vi "Get Result.vi"(8 "error in (no error)":errorcluster, 11 "LR-700 in":refnum<class "Linear Research.lvclass">) -> (0 "error out":errorcluster, 2 "Mag Lab Result.lvclass":refnum<class "Mag Lab Result.lvclass">, 3 "LR-700 out":refnum<class "Linear Research.lvclass">)   [LabVIEW 2015, in "Linear Research.lvclass"]
uses:
  Linear Research.lvclass
  Mag Lab Result/Mag Lab Result.lvclass
  Linear Research Parameters.ctl
  Mag Lab Hardware.lvclass/Mag Lab Hardware.ctl
  Mag Lab Root/Mag Lab Root.lvclass/Mag Lab Root.ctl
  Linear Research.lvclass/Linear Research.ctl
  Mag Lab Result/Mag Lab Result.lvclass/Mag Lab Result.ctl
  Mag Lab Properties/Mag Lab Parameters.lvclass
  Mag Lab Hardware.lvclass
  Mag Lab Error Handler/Mag Lab Error Handler.lvclass
  Mag Lab Root/Mag Lab Root.lvclass
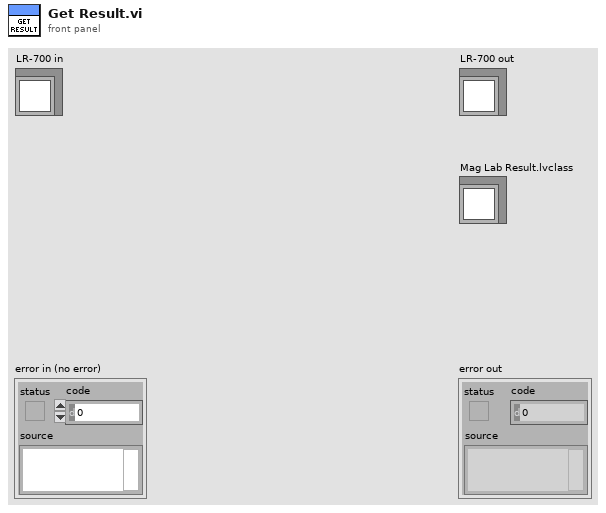
[diagram p1: front panel]
types:
  T1 = typedef "Linear Research Parameters.ctl" = cluster{"Scan  Channels":i32[], "Merge scan with":string}
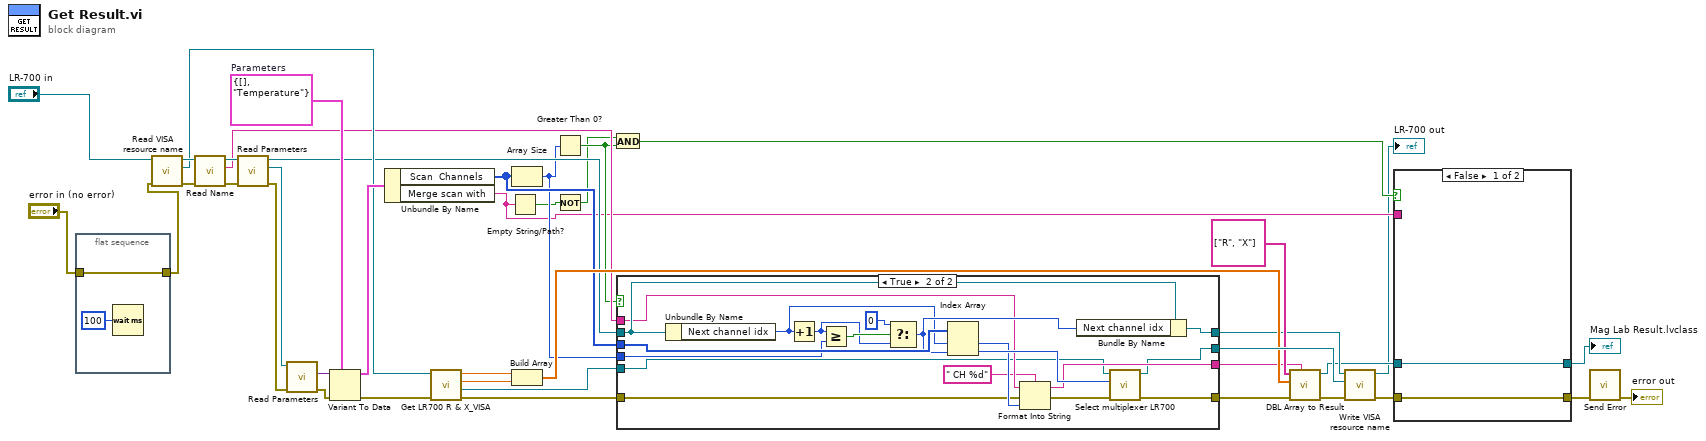
[diagram p0: block diagram]
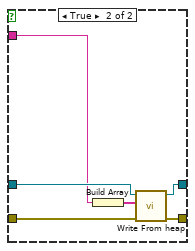
[diagram p2: hidden frame]
diagram:
  w37 = T1 {"Scan  Channels"=[], "Merge scan with"="Temperature"}  # Parameters
  n1 = flat-sequence {
    tunnel: "error in (no error)" -> [w43]
    tunnel: [w43] -> w1
    frame #0 {
      n2 = Wait (ms)(milliseconds to wait=u32 100) -> ()  [unwired: 1 out]
    }
  }
  n3 = call "Read VISA resource name.vi"("error in (no error)"=w1, "Mag Lab Hardware in"="LR-700 in") -> ("error out"=w40:errorcluster, "VISA resource name"=w28:refnum<visa-resource-name>, "Mag Lab Hardware out"=w41:refnum<class "Linear Research.lvclass">)  [unwired: 7 in]
  n4 = call "Read Name.vi"("error in (no error)"=w40, "Mag Lab Root in"=w41) -> ("error out"=w32:errorcluster, "Name"=w19:string, "Mag Lab Root out"=w31:refnum<class "Linear Research.lvclass">)  [unwired: 7 in]
  n5 = call-dynamic "Read Parameters.vi"("error in (no error)"=w32, "Mag Lab Root in"=w31) -> ("error out"=w34:errorcluster, "Mag Lab Parameters.lvclass"=w36:refnum<class "Mag Lab Parameters.lvclass">, "Mag Lab Root out"=w22:refnum<class "Linear Research.lvclass">)  [unwired: 7 in]
  n6 = call-dynamic "Read Parameters.vi"("error in (no error)"=w34, "Mag Lab Parameters in"=w36) -> ("error out"=w33:errorcluster, "Parameters"=w35:variant)  [unwired: 7 in, 1 out]
  n7 = Variant To Data(error in=w33, type=w37, Variant=w35) -> (data=w30:T1, error out=w5:errorcluster)
  n8 = Unbundle By Name(w30) -> ("Scan  Channels"=w21:i32[], "Merge scan with"=w9:string)
  n9 = call "Get LR700 R & X_VISA.vi"("error in (no error)"=w5, "VISA resource name"=w28) -> ("error out"=w17:errorcluster, "VISA resource name out"=w27:refnum<visa-resource-name>, "X"=w25:dbl, "Resistance"=w26:dbl)  [unwired: 2 in]
  n10 = Empty String/Path?(string/path=w9) -> (empty?=w6:bool)
  n11 = Array Size(array=w21) -> (size(s)=w20:i32)
  n12 = Build Array(w26, w25) -> (w24:dbl[])
  n13 = Greater Than 0?(x=w20) -> (x > 0?=w13:bool)
  n14 = Not(x=w6) -> (.not. x?=w7:bool)
  n15 = And(x=w7, y=w13) -> (x .and. y?=w8:bool)
  n16 = case shown="True" w13 {
    tunnel: w27 -> [w47 w49]
    tunnel: [w47 w48] -> w29
    tunnel: w22 -> [w44 w61]
    tunnel: w21 -> [_ w66]
    tunnel: w20 -> [_ w65]
    tunnel: w19 -> [w46 w56]
    tunnel: [w46 w54] -> w18
    tunnel: w17 -> [w45 w52]
    tunnel: [w45 w51] -> w16
    tunnel: [w44 w50] -> w15
    frame False {
    }
    frame True {
      n17 = Unbundle By Name(w61) -> ("Next channel idx"=w59:i32)
      n18 = Increment(x=w59) -> (x+1=w62:i32)
      n19 = Greater Or Equal?(x=w62, y=w65) -> (x >= y?=w64:bool)
      n20 = Select(t=0, s=w64, f=w62) -> (s? t:f=w60:i32)
      n21 = Index Array(array=w66, index #1=w59, index #2=w60) -> (element #1=w57:i32, element #2=w58:i32)
      n22 = Format Into String(format string=" CH %d", initial string=w56, error in=w52, w57) -> (resulting string=w54:string, error out=w53:errorcluster)
      n23 = Bundle By Name(cluster=w61, "Next channel idx"=w60) -> (w50:refnum<class "Linear Research.lvclass">)
      n24 = call "Select multiplexer LR700.vi"("error in"=w53, "Sensor <01-99>"=w58, "VISA Resource Name"=w49) -> ("error out"=w51:errorcluster, "VISA Resource Name Out"=w48:refnum<visa-resource-name>)  [unwired: 7 out]
    }
  }
  n25 = call "DBL Array to Result.vi"("Result name"=w18, "error in (no error)"=w16, "Data"=w24, "Channel Names"=string[] ["R", "X"]) -> ("error out"=w14:errorcluster, "Mag Lab Result out"=w12:refnum<class "Mag Lab Result.lvclass">)  [unwired: 6 in]
  n26 = call "Write VISA resource name.vi"("error in (no error)"=w14, "VISA resource name"=w29, "Mag Lab Hardware in"=w15) -> ("error out"=w11:errorcluster, "Mag Lab Hardware out"=→"LR-700 out":refnum<class "Linear Research.lvclass">)  [unwired: 7 in]
  n27 = case shown="False" w8 {
    tunnel: w12 -> [w68 w74]
    tunnel: w9 -> [_ w73]
    tunnel: w11 -> [w67 w71]
    tunnel: [w68 w70] -> w10
    tunnel: [w67 w69] -> w4
    frame False {
    }
    frame True {
      n28 = Build Array(w73) -> (w72:string[])
      n29 = call "Write From heap.vi"("error in (no error)"=w71, "From heap"=w72, "Mag Lab Result in"=w74) -> ("error out"=w69:errorcluster, "Mag Lab Result out"=w70:refnum<class "Mag Lab Result.lvclass">)  [unwired: 7 in]
    }
  }
  "Mag Lab Result.lvclass" <- w10
  n30 = call "Send Error.vi"("error in (no error)"=w4) -> ("error out"=→"error out":errorcluster)  [unwired: 9 in, 1 out]
